vi "HAL Test.vi"() -> ()   [LabVIEW 2020, in "LAF2024Q2.lvlib"]
uses:
  LAF2024Q2.lvlib
  PsuVisaSim/PsuVisaSim.lvclass
  C:/dev/lv20CE/LAF2024Q2/LAF2024Q2/PowerSupplyVisa/PowerSupplyVisa.lvclass
  Keithley230X/Keithley230X.lvclass
  PowerSupply/PowerSupply.lvclass
panel:
  out "error out":errorcluster
  in  "Sim?":bool
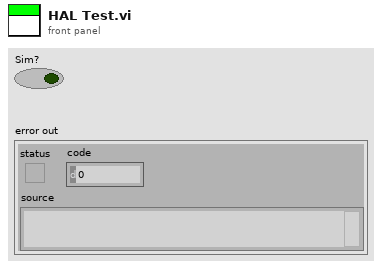
[diagram p1: front panel]
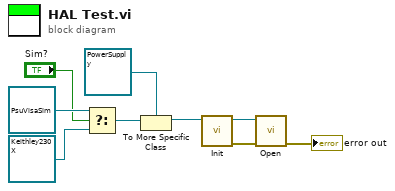
[diagram p0: block diagram]
diagram:
  n1 = Select(t=refnum<class "PsuVisaSim.lvclass"> refnum ("LAF2024Q2.lvlib:PsuVisaSim.lvclass"), s="Sim?", f=refnum<class "Keithley230X.lvclass"> refnum ("LAF2024Q2.lvlib:Keithley230X.lvclass")) -> (s? t:f=w6:refnum<class "PowerSupplyVisa.lvclass">)
  n2 = To More Specific Class(target class=refnum<class "PowerSupply.lvclass"> refnum ("LAF2024Q2.lvlib:PowerSupply.lvclass"), reference=w6) -> (specific class reference=w2:refnum<class "PowerSupply.lvclass">)  [unwired: 1 in, 1 out]
  n3 = call-dynamic "Init.vi"("PowerSupply in"=w2) -> ("error out"=w4:errorcluster, "PowerSupply out"=w5:refnum<class "PowerSupply.lvclass">)  [unwired: 9 in]
  n4 = call-dynamic "Open.vi"("error in (no error)"=w4, "PowerSupply in"=w5) -> ("error out"=→"error out":errorcluster)  [unwired: 8 in, 1 out]
